vi "Jeffress_model_v010.vi"() -> ()   [LabVIEW 2019]
panel:
  out "Index":string
  out "new picture":picture
  in  "stop":bool
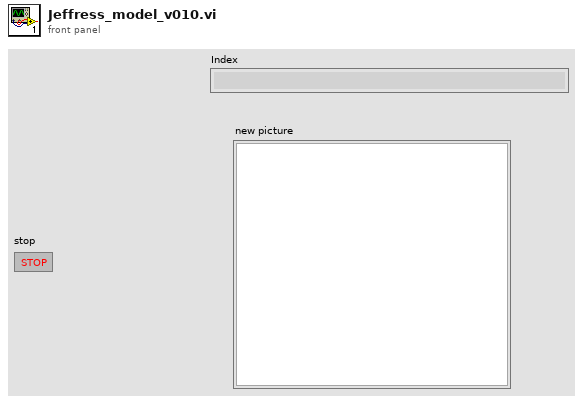
[diagram p1: front panel]
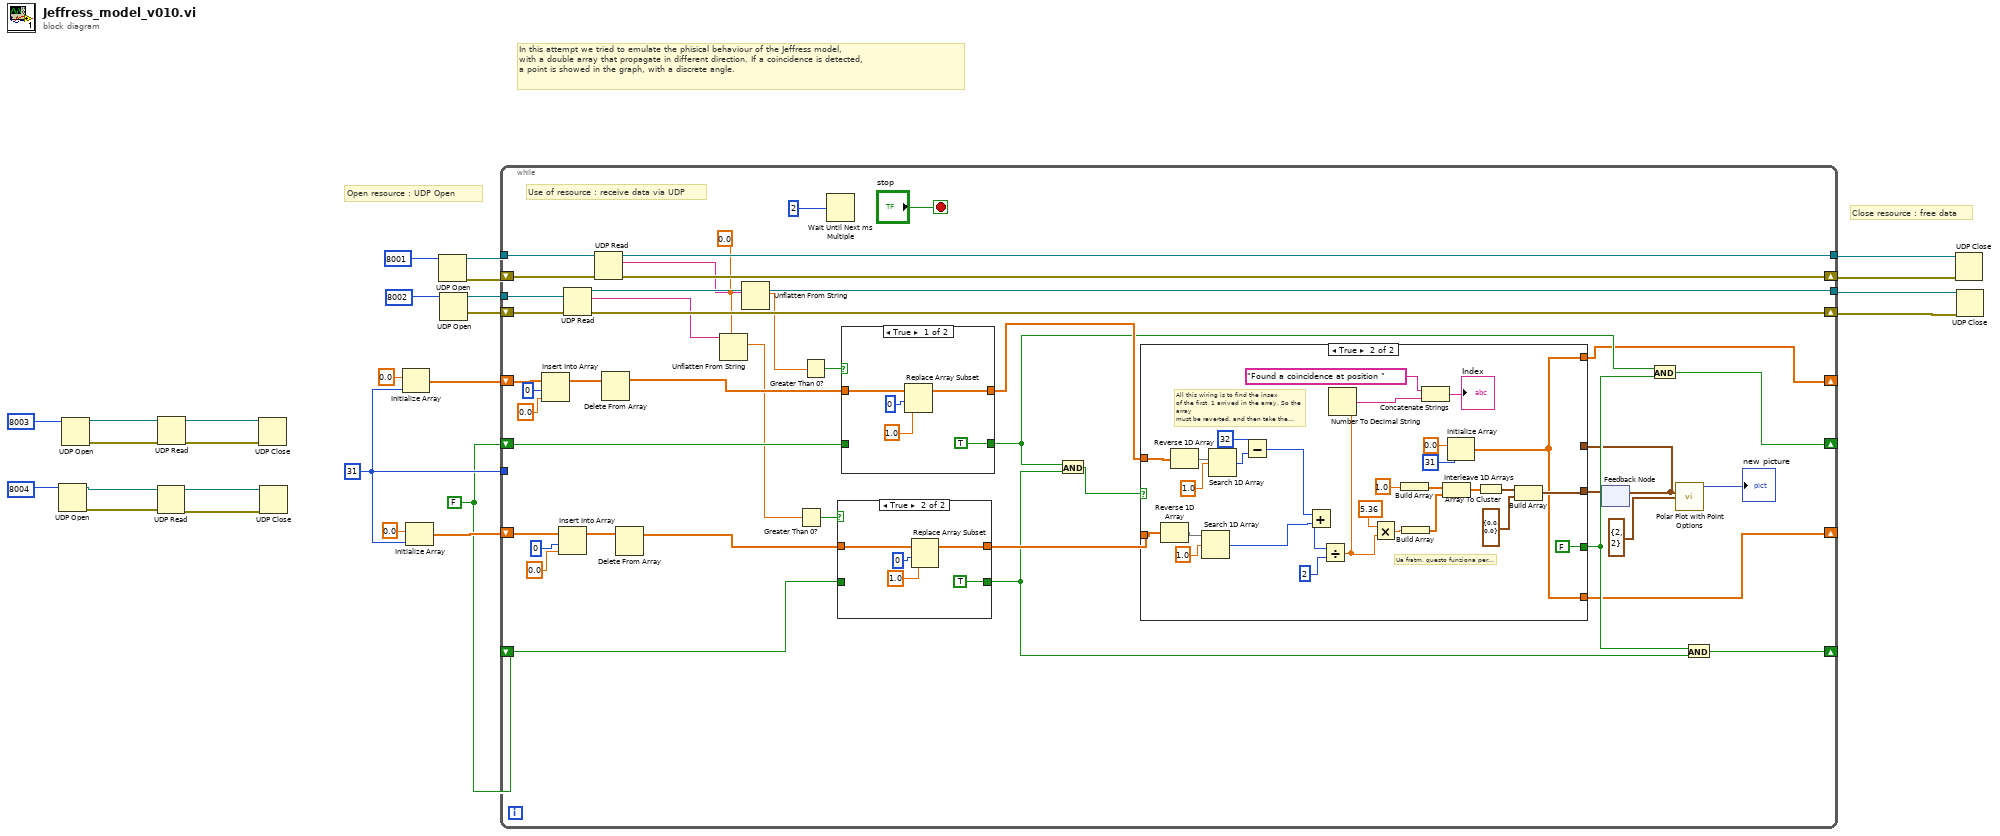
[diagram p0: block diagram]
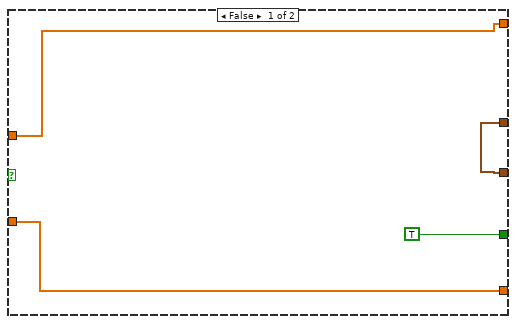
[diagram p2: hidden frame]
diagram:
  w11 = FALSE
  w12 = 31 ("dimension size")
  # "In this attempt we tried to emulate the phisical behaviour of the Jeffress model,\nwith a double array that propagate in different direction. If a coincidence is detected,\na point is showed in the graph, with a discrete angle."
  # "Close resource : free data"
  # "Open resource : UDP Open"
  n1 = UDP Open(11:u16 8004) -> (port=w6:refnum<k16>, 0:w5:errorcluster)  [unwired: 4 in, 1 out]
  n2 = UDP Open(11:u16 8003) -> (port=w8:refnum<k16>, 0:w7:errorcluster)  [unwired: 4 in, 1 out]
  n3 = UDP Read(connection ID=w6, 8:w5) -> (error out=w1:errorcluster, 3:w2:refnum<k16>)  [unwired: 2 in, 3 out]
  n4 = UDP Read(connection ID=w8, 8:w7) -> (error out=w3:errorcluster, 3:w4:refnum<k16>)  [unwired: 2 in, 3 out]
  n5 = UDP Close(connection ID=w4, 8:w3) -> ()  [unwired: 2 out]
  n6 = UDP Close(connection ID=w2, 8:w1) -> ()  [unwired: 2 out]
  n7 = Initialize Array(0.0 ("element"), w12) -> (w15:dbl[])
  n8 = Initialize Array(0.0 ("element"), w12) -> (w13:dbl[])
  n9 = UDP Open(11:u16 8001) -> (port=w24:refnum<k16>, 0:w26:errorcluster)  [unwired: 4 in, 1 out]
  n10 = UDP Open(11:u16 8002) -> (port=w20:refnum<k16>, 0:w19:errorcluster)  [unwired: 4 in, 1 out]
  n11 = while {
    tunnel: w24 -> [w65]
    tunnel: [w64] -> w23
    shift-right: [w67] -> w25
    shift-left: w26 -> [w66]
    tunnel: w20 -> [w61]
    shift-right: [w58] -> w18
    shift-left: w19 -> [w60]
    tunnel: [w59] -> w17
    shift-right: [w37] -> _
    shift-left: w15 -> [w57]
    shift-right: [w36] -> _
    shift-left: w13 -> [w49]
    tunnel: w12 -> [_]
    shift-right: [w39] -> _
    shift-left: w11 -> [w44]
    shift-right: [w38] -> _
    shift-left: w11 -> [w43]
    stop <- "stop" stop-if-true
    w31 = 0.0
    # "Use of resource : receive data via UDP"
    n12 = Insert Into Array(array=w57, index=0, new element=0.0 ("new element/subarray")) -> (w54:dbl[])
    n13 = Insert Into Array(array=w49, index=0, new element=0.0 ("new element/subarray")) -> (w50:dbl[])
    n14 = UDP Read(connection ID=w61, 8:w60) -> (data out=w32:string, error out=w58:errorcluster, 3:w59:refnum<k16>)  [unwired: 2 in, 2 out]
    n15 = UDP Read(connection ID=w65, 8:w66) -> (data out=w33:string, error out=w67:errorcluster, 3:w64:refnum<k16>)  [unwired: 2 in, 2 out]
    n16 = Delete From Array(array=w54) -> (array with subset deleted=w53:dbl[])  [unwired: 2 in, 1 out]
    n17 = Delete From Array(array=w50) -> (array with subset deleted=w48:dbl[])  [unwired: 2 in, 1 out]
    n18 = Unflatten From String(type=w31, binary string=w32) -> (value=w28:dbl)  [unwired: 3 in, 2 out]
    n19 = Unflatten From String(type=w31, binary string=w33) -> (value=w29:dbl)  [unwired: 3 in, 2 out]
    n20 = Greater Than 0?(x=w28) -> (x > 0?=w27:bool)
    n21 = Greater Than 0?(x=w29) -> (x > 0?=w30:bool)
    n22 = Wait Until Next ms Multiple(millisecond multiple=u32 2) -> ()  [unwired: 1 out]
    n23 = case shown="True" w27 {
      tunnel: [w104 w107] -> w45
      tunnel: w48 -> [w104 w106]
      tunnel: [w103 TRUE] -> w42
      tunnel: w43 -> [w103 _]
      frame False {
      }
      frame True {
        n24 = Replace Array Subset(array=w106, new element=1.0 ("new element/subarray"), index=0) -> (w107:dbl[])
      }
    }
    n25 = case shown="True" w30 {
      tunnel: [w112 w116] -> w46
      tunnel: w53 -> [w111 w116]
      tunnel: [TRUE w115] -> w40
      tunnel: w44 -> [_ w115]
      frame True {
        n26 = Replace Array Subset(array=w111, new element=1.0 ("new element/subarray"), index=0) -> (w112:dbl[])
      }
      frame False {
      }
    }
    n27 = And(x=w40, y=w42) -> (x .and. y?=w47:bool)
    n28 = feedback #1() -> (w34:cluster{"[0]":dbl, "[1]":dbl}[])  [unwired: 1 in]
    n29 = case shown="True" w47 {
      tunnel: [w70 w83] -> w35
      tunnel: w46 -> [w72 w94]
      tunnel: w45 -> [w71 w77]
      tunnel: [TRUE FALSE] -> w41
      tunnel: [w72 w79] -> w37
      tunnel: [w71 w79] -> w36
      tunnel: w34 -> [w70 _]
      frame False {
      }
      frame True {
        # "Ua fratm, questo funziona per forza"
        # "All this wiring is to find the insex\nof the first  1 arrived in the array. So the array \nmust be reverted, and then take the original \nindex."
        n30 = Reverse 1D Array(array=w77) -> (reversed array=w78:dbl[])
        n31 = Reverse 1D Array(array=w94) -> (reversed array=w93:dbl[])
        n32 = Search 1D Array(1D array=w78, element=1.0) -> (index of element=w75:i32)  [unwired: 1 in]
        n33 = Search 1D Array(1D array=w93, element=1.0) -> (index of element=w89:i32)  [unwired: 1 in]
        n34 = Subtract(x=32, y=w89) -> (x-y=w74:i32)
        n35 = Add(x=w74, y=w75) -> (x+y=w97:i32)
        n36 = Divide(x=w97, y=2) -> (x/y=w95:dbl)
        n37 = Number To Decimal String(number=w95) -> (decimal integer string=w101:string)  [unwired: 1 in]
        n38 = Multiply(x=5.36, y=w95) -> (x*y=w102:dbl)
        n39 = Build Array(1.0) -> (w87:dbl[])
        n40 = Build Array(w102) -> (w86:dbl[])
        n41 = Concatenate Strings("Found a coincidence at position ", w101) -> (→"Index":string)
        n42 = Interleave 1D Arrays(w87, w86) -> (w85:dbl[])
        n43 = Initialize Array(0.0 ("element"), 31 ("dimension size")) -> (w79:dbl[])
        n44 = Array To Cluster(array=w85) -> (cluster=w84:cluster{"[0]":dbl, "[1]":dbl})
        n45 = Build Array(w84, cluster{"[0]":dbl, "[1]":dbl} {"[0]"=0.0, "[1]"=0.0} ("element")) -> (w83:cluster{"[0]":dbl, "[1]":dbl}[])
      }
    }
    n46 = feedback-in #1(w35) -> ()
    n47 = And(x=w40, y=w41) -> (x .and. y?=w39:bool)
    n48 = call <vilib>:"Polar Plot with Point Options.vi"("data array [mag, phase (deg)]"=w34, "top left point(0, 0)"=cluster{"x":i16, "y":i16} {"x"=2, "y"=2}) -> ("new picture"=→"new picture":picture)  [unwired: 13 in]
    n49 = And(x=w41, y=w42) -> (x .and. y?=w38:bool)
  }
  n50 = UDP Close(connection ID=w23, 8:w25) -> ()  [unwired: 2 out]
  n51 = UDP Close(connection ID=w17, 8:w18) -> ()  [unwired: 2 out]
